vi "Run_Lock_In.vi"(6 "Reference Signal Sampling Rate":dbl, 8 "LP Filter Cuttoff Freq":dbl, 9 "Output in Polar?":bool=TRUE, 10 "error in (no error)":errorcluster, 11 "Working Directory":string) -> (1 "standard output":string, 2 "error out":errorcluster, 3 "standard error":string)   [LabVIEW 2012]
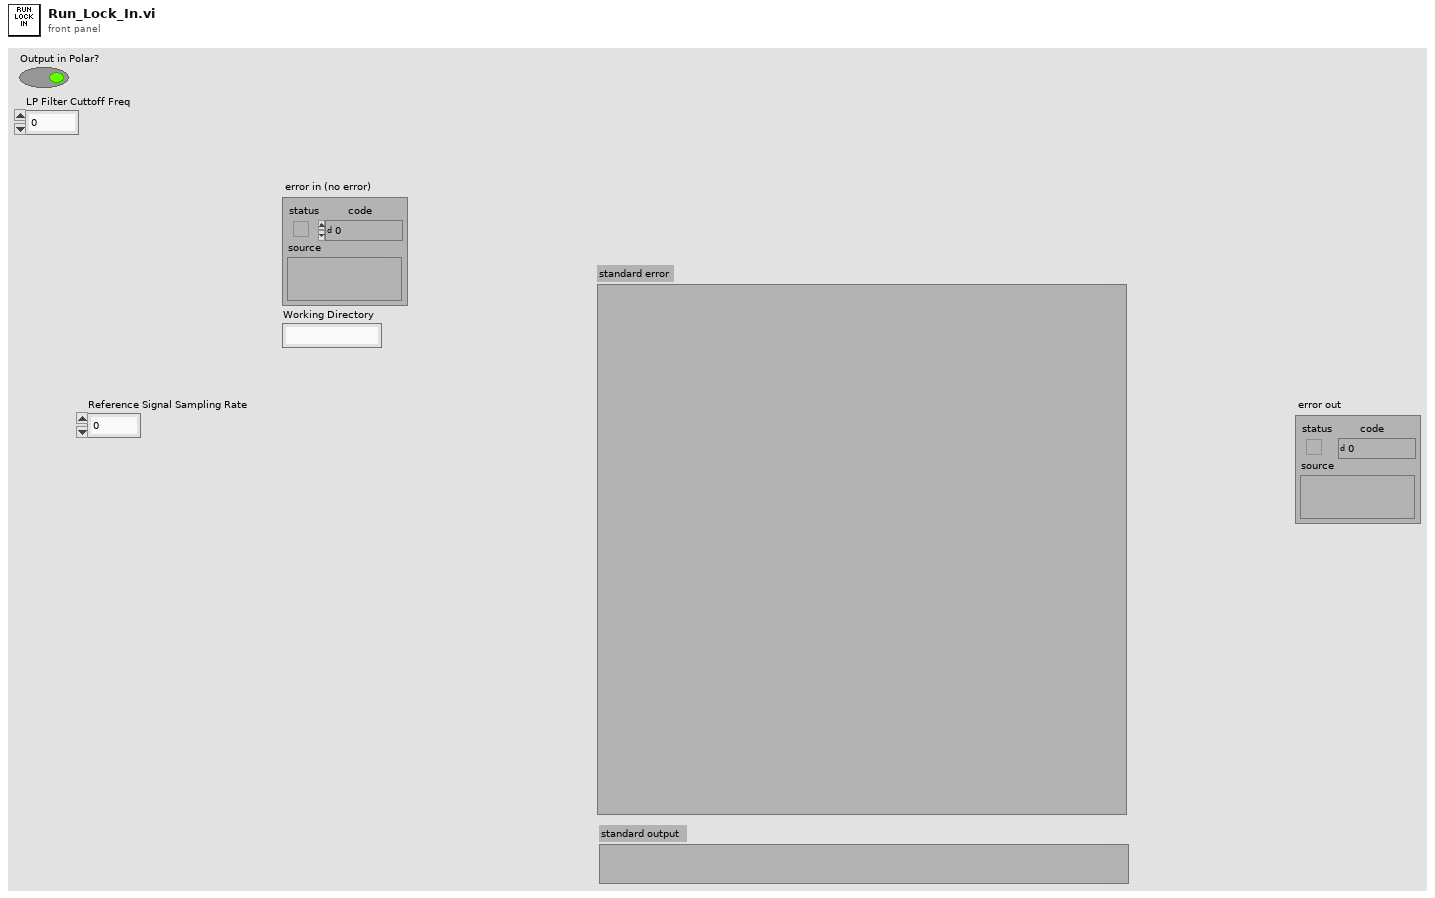
[diagram p1: front panel]
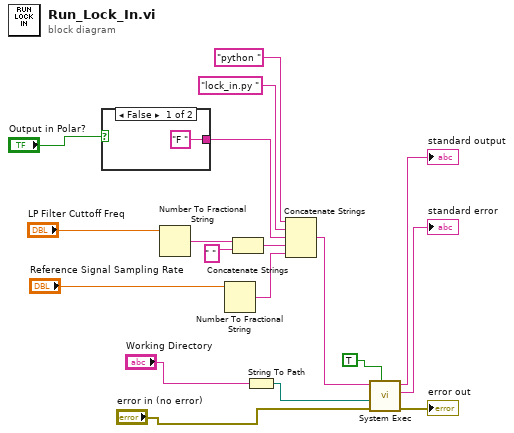
[diagram p0: block diagram]
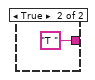
[diagram p2: hidden frame]
diagram:
  n1 = case shown="False" "Output in Polar?" {
    tunnel: ["F " "T "] -> w8
    frame False {
    }
    frame True {
    }
  }
  n2 = Number To Fractional String(number="LP Filter Cuttoff Freq") -> (F-format string=w5:string)  [unwired: 3 in]
  n3 = Number To Fractional String(number="Reference Signal Sampling Rate") -> (F-format string=w1:string)  [unwired: 3 in]
  n4 = Concatenate Strings(w5, " " ("string")) -> (w3:string)
  n5 = String To Path(string="Working Directory") -> (path=w11:path)
  n6 = Concatenate Strings("python " ("string"), "lock_in.py " ("string"), w8, w3, w1) -> (w12:string)
  n7 = call <vilib>:"System Exec.vi"("wait until completion? (T)"=TRUE, "error in (no error)"="error in (no error)", "working directory"=w11, "command line"=w12) -> ("error out"=→"error out":errorcluster, "standard error"=→"standard error":string, "standard output"=→"standard output":string)  [unwired: 4 in, 1 out]
